vi "Select Calculation Dialog.vi"(8 "error in (no error)":errorcluster, 11 "Node Ptr":u64 format="%.0x") -> (0 "error out":errorcluster)   [LabVIEW 2015, in "Waveform-Processing-Custom-Device System Explorer.lvlib"]
uses:
  Waveform-Processing-Custom-Device System Explorer.lvlib
panel:
  in  "OK Button":bool
  in  "Select a calculation :":u16(ring)
  in  "Tag":string
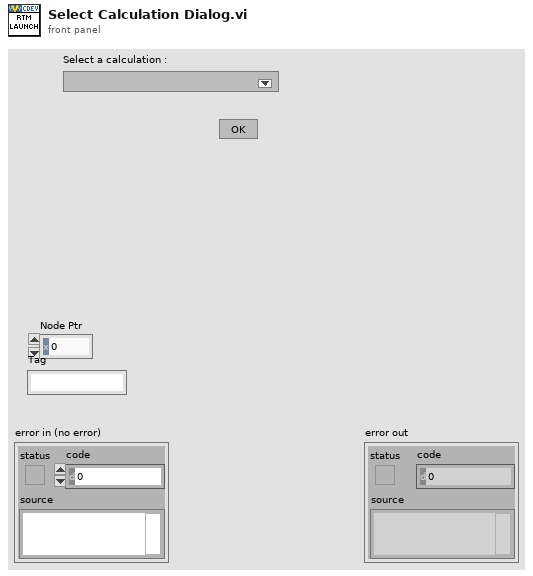
[diagram p1: front panel]
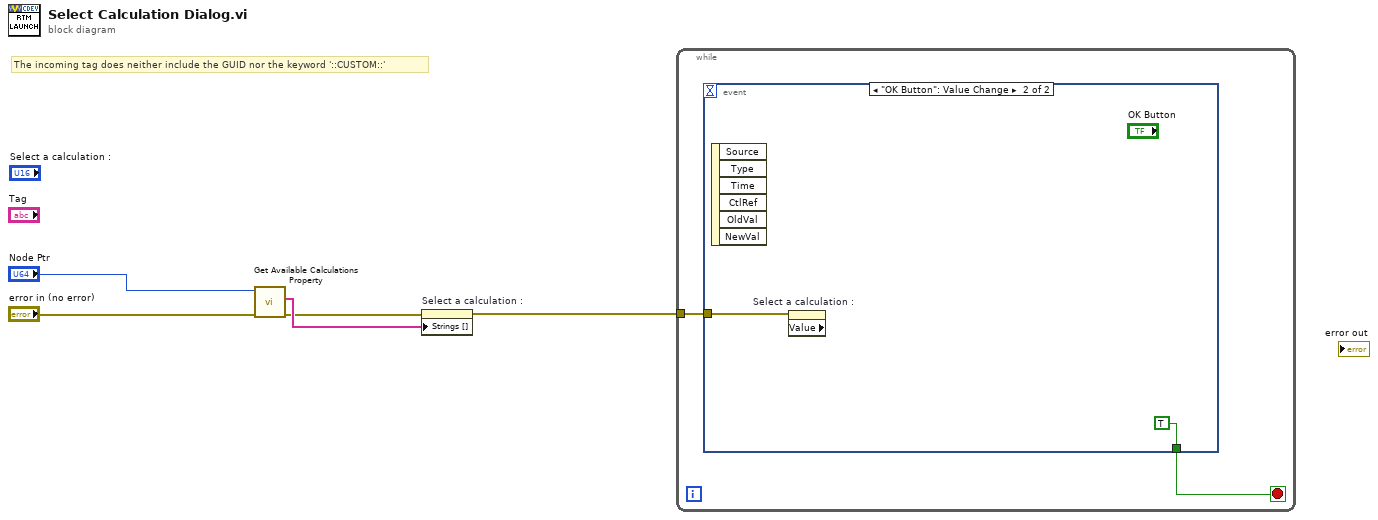
[diagram p0: block diagram]
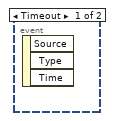
[diagram p2: hidden frame]
diagram:
  # "The incoming tag does neither include the GUID nor the keyword '::CUSTOM::'"
  n1 = call "Get Available Calculations Property.vi"("error in (no error)"="error in (no error)", "Device Item Ref"="Node Ptr") -> ("error in (no error) out"=w2:errorcluster, "Available Calculations"=w3:string[])  [unwired: 7 in, 1 out]
  n2 = property on="Select a calculation :" class="Ring (strict)"(error in=w2, "Strings []"=w3) -> (error out=w1:errorcluster)  [unwired: 1 in, 1 out]
  n3 = while {
    tunnel: w1 -> [w7]
    stop <- w6 stop-if-true
    n4 = event shown="[1] \"OK Button\": Value Change" {
      selector: _ -> [_ _]
      dyn-events: _ -> [_ _]
      timeout: _ -> [_ _]
      tunnel: w7 -> [_ w9]
      tunnel: [_ TRUE] -> w6
      event Timeout {
        n5 = event-data() -> ()  [unwired: 1 in, 3 out]
      }
      event "OK Button": Value Change {
        n6 = event-data() -> ()  [unwired: 1 in, 6 out]
        n7 = property on="Select a calculation :" class="Ring (strict)" props=["Value"](error in=w9) -> ()  [unwired: 1 in, 3 out]
      }
    }
  }
